vi "SynapseAPI-Get Mode.vi"(0 "URL":string="http://localhost:24414", 11 "error in (no error)":errorcluster) -> (8 "mode":T1, 15 "error out":errorcluster)   [LabVIEW 2020]
uses:
  SynapseAPI-Mode.ctl
  <vilib>/httpClient/LabVIEWHTTPClient.lvlib
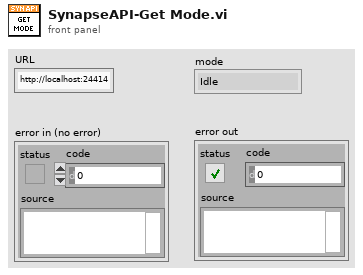
[diagram p1: front panel]
types:
  T1 = typedef "SynapseAPI-Mode.ctl" = enum16{"Idle", "Standby", "Preview", "Record"}
  T2 = typedef "LabVIEWHTTPClient.lvlib/ClientHandle.ctl" = refnum<k1>
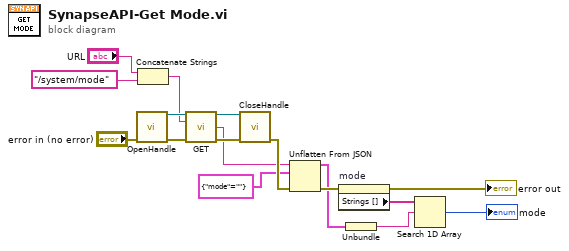
[diagram p0: block diagram]
diagram:
  n1 = call <vilib>:"OpenHandle.vi"("error in (no error)"="error in (no error)") -> ("client handle out"=w14:T2, "error out"=w13:errorcluster)  [unwired: 13 in]
  n2 = Concatenate Strings("URL", "/system/mode") -> (w2:string)
  n3 = call <vilib>:"GET.vi"("client handle"=w14, "url"=w2, "error in (no error)"=w13) -> ("client handle out"=w16:T2, "body"=w10:string, "error out"=w17:errorcluster)  [unwired: 9 in, 1 out]
  n4 = call <vilib>:"CloseHandle.vi"("client handle"=w16, "error in (no error)"=w17) -> ("error out"=w12:errorcluster)  [unwired: 13 in]
  n5 = Unflatten From JSON(JSON string=w10, type and defaults=cluster{"mode":string} {"mode"=""} ("Cluster"), error in (no error)=w12) -> (value=w6:cluster{"mode":string}, error out=w8:errorcluster)  [unwired: 4 in]
  n6 = property on="mode" class="Enum (strict)"(error in=w8) -> (error out=→"error out":errorcluster, "Strings []"=w7:string[])  [unwired: 1 in, 1 out]
  n7 = Unbundle(w6) -> ("mode"=w5:string)
  n8 = Search 1D Array(1D array=w7, element=w5) -> (index of element=→"mode":i32)  [unwired: 1 in]
